vi "OAT Get Even Angle Reference (N Channels).vi"(0 "scaled signals [EU]":waveform(dbl)[](array[waveform]), 1 "reference output mode":T2(ring), 2 "reset? (F)":bool, 5 "speed profile":T1 {"speed [RPM]" format="%.2f"; "time [s]" format="%.2f"}, 7 "pulse/revolution (1)":i32=1, 9 "# of revs in reference":i32=1, 11 "error in (no error)":errorcluster, 12 "max order (auto)":dbl, 13 "remove DC? (F)":bool) -> (4 "even-angle references":cluster{"r0":dbl, "dr":dbl, "Y":dbl[]}[](array[cluster]) {"r0" format="%.2p"; "dr" format="%.2p"; "Y" format="%.2f"}, 14 "actual max order":dbl, 15 "error out":errorcluster)   [LabVIEW 2017, in "SoundVib_RefDataProcess.lvlib"]
doc: "Computes the even-angle reference of the <B>scaled signal [EU]</B>. The output reference is the even-angle spaced signal with a constant number of samples per revolution. Wire data to the <B>scaled signal [EU]</B> input to determine the polymorphic instance to use or manually select the instance."
uses:
  <vilib>/addons/Sound and Vibration/Order Analysis/Referece Data Processing/SoundVib_RefDataProcess.lvlib
  <vilib>/addons/Sound and Vibration/Order Analysis/Tach Process/SubVIs/speed profile.ctl
  <vilib>/addons/_NISVFA/_Shared subVIs/Common/svc_Check for Waveform Parameter Continuity (no state).vi
  <vilib>/addons/_NISVFA/_Shared subVIs/Common/svc_Get SV Channel Info.vi
  <vilib>/addons/Sound and Vibration/Order Analysis/Utility/OAT AC DC Separation (N Channels).vi
  <vilib>/addons/Sound and Vibration/Order Analysis/Resample Order Tracking/OAT Convert to Even Angle Signal (N Channels).vi
  <vilib>/addons/_NISVFA/_Shared subVIs/Common/svc_Engineering Units to Unit Label.vi
  <vilib>/addons/_NISVFA/_Shared subVIs/Common/svc_Unit Label to Engineering Units.vi
  <vilib>/addons/Sound and Vibration/Order Analysis/Resample Order Tracking/SoundVib_Resampling.lvlib
  <vilib>/addons/Sound and Vibration/Order Analysis/Resample Order Tracking/SoundVib_OrderTracking.lvlib
  <vilib>/addons/Sound and Vibration/Order Analysis/Utility/SoundVib_OAUtility.lvlib
  <vilib>/addons/Sound and Vibration/Order Analysis/Tach Process/SoundVib_TachProcess.lvlib
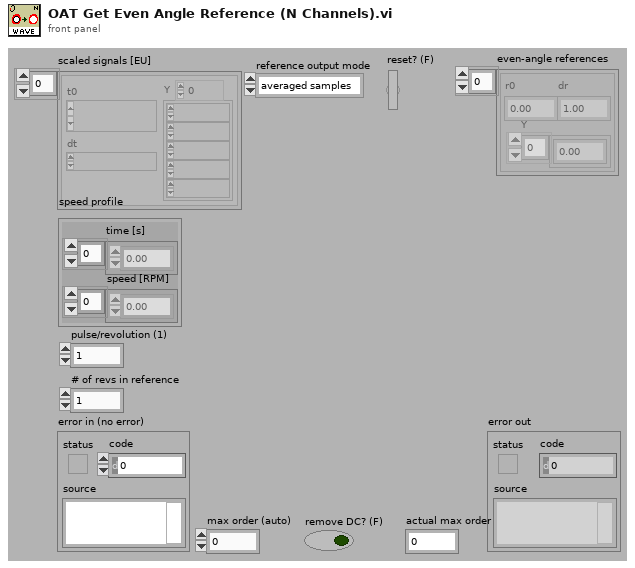
[diagram p1: front panel]
types:
  T1 = typedef "SoundVib_TachProcess.lvlib/speed profile.ctl" = cluster{"time [s]":dbl[], "speed [RPM]":dbl[]}
  T2 = enum16{"averaged samples", "initial samples", "final samples"}
  T3 = cluster{"dt equal":bool, "array length equal":bool, "number channels change":bool}
  T4 = cluster{"dt":bool, "t0 continuity":bool, "array length":bool, "channel info":bool, "name":bool}
  T5 = cluster{"r0":dbl, "dr":dbl, "reference data":dbl[]}[]
  T6 = typedef "svc_Resampled Channel Info.ctl" = cluster{"channel name":string, "description":string, " channel info":T7}
  T7 = typedef "svc_Channel Info.ctl" = cluster{"sensor sensitivity":dbl, "engineering units":T8, "dB reference":dbl, "custom label":string, "weighting filter":T9, "pregain":dbl}
  T8 = typedef "svc_Engineering Units Text Ring.ctl" = u16
  T9 = typedef "svc_Weighting Filter Text Ring.ctl" = u16
  T10 = typedef "OAT Position Info.ctl" = cluster{"positions [s]":dbl[], "samples/rev":dbl}
  T11 = cluster{"r0":dbl, "dr":dbl, "reference data":dbl[]}
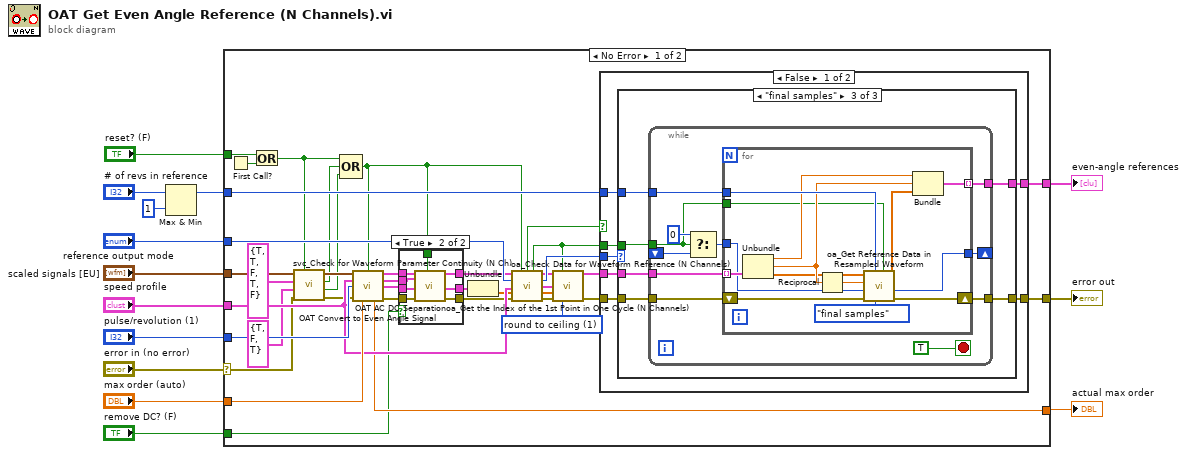
[diagram p0: block diagram]
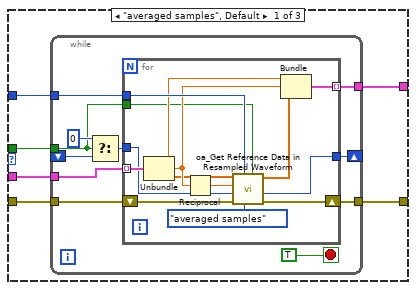
[diagram p3: hidden frame]
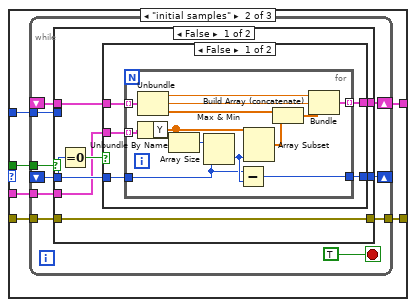
[diagram p4: hidden frame]
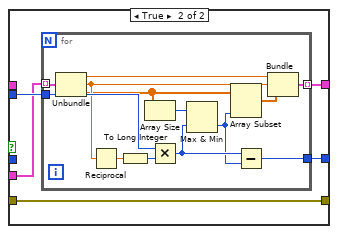
[diagram p6: hidden frame]
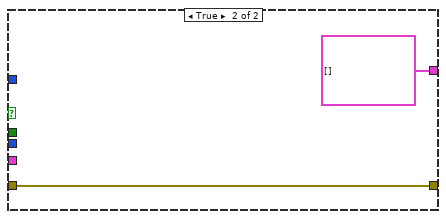
[diagram p7: hidden frame]
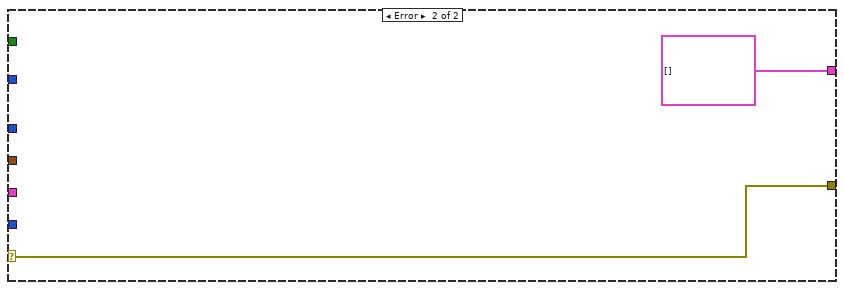
[diagram p8: hidden frame]
diagram:
  n1 = Max & Min(x="# of revs in reference", y=1) -> (max(x,y)=w9:i32)  [unwired: 1 out]
  n2 = case shown="No Error" "error in (no error)" {
    selector: "error in (no error)" -> [w22 w198]
    tunnel: "reference output mode" -> [w53 _]
    tunnel: [w52 T5 []] -> w12
    tunnel: [w51 w198] -> w11
    tunnel: w9 -> [w47 _]
    tunnel: "scaled signals [EU]" -> [w24 _]
    tunnel: "pulse/revolution (1)" -> [w44 _]
    tunnel: "max order (auto)" -> [w43 _]
    tunnel: "speed profile" -> [w42 _]
    tunnel: [w37 _] -> w3
    tunnel: "reset? (F)" -> [w36 _]
    tunnel: "remove DC? (F)" -> [w28 _]
    frame No Error {
      w33 = u16 1 items=["round to nearest", "round to ceiling"] ("index mode")
      n3 = First Call?() -> (First Call?: T/F=w38:bool)
      n4 = Or(x=w36, y=w38) -> (x .or. y?=w20:bool)
      n5 = call <vilib>:"svc_Check for Waveform Parameter Continuity (N Ch).vi"("restart averaging (F)"=w20, "error in (no error)"=w22, "checks for multichannel parameters"=T3 {"dt equal"=TRUE, "array length equal"=FALSE, "number channels change"=TRUE}, "checks for channel parameter change"=T4 {"dt"=TRUE, "t0 continuity"=TRUE, "array length"=FALSE, "channel info"=TRUE, "name"=FALSE}, "scaled signal(s)"=w24) -> ("error out"=w21:errorcluster, "multichannel parameter changed"=w17:bool, "waveform parameter changed"=w18:bool, "dup scaled signal(s)"=w23:waveform(dbl)[])  [unwired: 3 out]
      n6 = Compound Arithmetic op=OR(w20, w18, w17) -> (w19:bool)
      n7 = call-poly <vilib>:"OAT Convert to Even Angle Signal.vi"("scaled signals [EU]"=w23, "reset? (F)"=w19, "speed profile"=w42, "pulse/revolution (1)"=w44, "error in (no error)"=w21, "max order (auto)"=w43) -> ("even-angle signals"=w32:cluster{"r0":dbl, "dr":dbl, "Y":dbl[]}[], "even-angle channel info"=w29:T6[], "even-angle position info"=w26:T10, "actual max order"=w37:dbl, "error out"=w25:errorcluster)  [unwired: 5 in]
      n8 = case shown="True" w28 {
        tunnel: w32 -> [w56 w64]
        tunnel: [w56 w59] -> w31
        tunnel: w25 -> [w55 w63]
        tunnel: [w55 w62] -> w30
        tunnel: w19 -> [_ w61]
        tunnel: w29 -> [_ w60]
        tunnel: w26 -> [w54 w58]
        tunnel: [w54 w57] -> w27
        frame False {
        }
        frame True {
          n9 = call-poly <vilib>:"OAT AC DC Separation.vi"("even-angle signals"=w64, "even-angle channel info"=w60, "position info"=w58, "error in (no error)"=w63, "reset? (F)"=w61) -> ("even-angle AC signals"=w59:cluster{"r0":dbl, "dr":dbl, "Y":dbl[]}[], "position info out"=w57:T10, "error out"=w62:errorcluster)  [unwired: 9 in, 3 out]
        }
      }
      n10 = Unbundle(w27) -> ("positions [s]"=w39:dbl[])  [unwired: 1 out]
      n11 = call <vilib>:"oa_Check Data for Waveform Reference (N Channels).vi"("resampled signal"=w31, "reset? (True)"=w19, "select reference data"=w53, "speed profile"=w42, "interpolated pulse positions"=w39, "error in (no error)"=w30) -> ("empty signal?"=w35:bool, "reset"=w34:bool, "resampled data out"=w46:cluster{"r0":dbl, "dr":dbl, "Y":dbl[]}[], "select reference dataout"=w50:T2, "speed profile out"=w49:T1, "interpolated pulse positions out"=w48:dbl[], "error out"=w45:errorcluster)  [unwired: 2 in, 1 out]
      n12 = call <vilib>:"oa_Get the Index of the 1st Point in One Cycle (N Channels).vi"("resampled signal"=w46, "reset? (True)"=w34, "speed profile"=w49, "interpolated pulse positions"=w48, "error in (no error)"=w45, "index mode"=w33) -> ("resampled signal out"=w40:cluster{"r0":dbl, "dr":dbl, "Y":dbl[]}[], "error out"=w41:errorcluster)  [unwired: 7 in, 1 out]
      n13 = case shown="False" w35 {
        tunnel: [w71 T5 []] -> w52
        tunnel: [w70 w196] -> w51
        tunnel: w34 -> [w69 _]
        tunnel: w50 -> [w68 _]
        tunnel: w47 -> [w67 _]
        tunnel: w41 -> [w66 w196]
        tunnel: w40 -> [w65 _]
        frame False {
          n14 = case shown="\"final samples\"" w68 {
            tunnel: w69 -> [w77 w108 w169]
            tunnel: w67 -> [w76 w107 w168]
            tunnel: [w75 w105 w166] -> w71
            tunnel: [w74 w106 w167] -> w70
            tunnel: w66 -> [w72 w104 w165]
            tunnel: w65 -> [w73 w103 w164]
            frame "averaged samples", Default {
              n15 = while {
                tunnel: w77 -> [w79]
                tunnel: w76 -> [w87]
                tunnel: [w86] -> w75
                shift-right: [w85] -> _
                shift-left: _ -> [w83]
                tunnel: [w84] -> w74
                tunnel: w73 -> [w80]
                tunnel: w72 -> [w78]
                stop <- TRUE stop-if-true
                n16 = Select(t=0, s=w79, f=w83) -> (s? t:f=w81:i32)
                n17 = for {
                  tunnel: w80 -> [w92] mode=indexing
                  tunnel: w87 -> [w102]
                  tunnel: [w98] -> w86 mode=indexing
                  tunnel: [w97] -> w85
                  shift-right: [w96] -> w84
                  shift-left: w78 -> [w101]
                  tunnel: w81 -> [w90]
                  tunnel: w79 -> [w89]
                  n18 = Unbundle(w92) -> ("r0"=w94:dbl, "dr"=w93:dbl, "Y"=w91:dbl[])
                  n19 = Reciprocal(x=w93) -> (1/x=w99:dbl)
                  n20 = call <vilib>:"oa_Get Reference Data in Resampled Waveform.vi"("reset? (True)"=w89, "select reference data"=T2."averaged samples", "# of revs in reference data"=w102, "error in (no error)"=w101, "last index"=w90, "pulse per rev"=w99, "Y"=w91) -> ("error out"=w96:errorcluster, "last index out"=w97:i32, "reference data"=w100:dbl[])  [unwired: 2 in]
                  n21 = Bundle("r0"=w94, "dr"=w93, "reference data"=w100) -> (w98:T11)  [unwired: 1 in]
                }
              }
            }
            frame "initial samples" {
              n22 = while {
                tunnel: w108 -> [w111]
                tunnel: w107 -> [w117]
                shift-right: [w116] -> w105
                shift-left: _ -> [w114]
                shift-right: [w115] -> _
                shift-left: _ -> [w113]
                tunnel: [w112] -> w106
                tunnel: w104 -> [w110]
                tunnel: w103 -> [w109]
                stop <- TRUE stop-if-true
                n23 = case shown="False" w111 {
                  tunnel: w110 -> [w120 w146]
                  tunnel: w117 -> [_ w150]
                  tunnel: [w121 w149] -> w116
                  tunnel: [w125 w148] -> w115
                  tunnel: w114 -> [w124 _]
                  tunnel: w113 -> [w123 _]
                  tunnel: [w120 w146] -> w112
                  tunnel: w109 -> [w119 w147]
                  frame False {
                    n24 = Equal To 0?(x=w123) -> (x = 0?=w122:bool)
                    n25 = case shown="False" w122 {
                      tunnel: [w130 w144] -> w125
                      tunnel: w124 -> [w129 w145]
                      tunnel: w123 -> [w128 w144]
                      tunnel: [w127 w145] -> w121
                      tunnel: w119 -> [w126 _]
                      frame False {
                        n26 = for {
                          tunnel: [w142] -> w130
                          tunnel: w129 -> [w140] mode=indexing
                          tunnel: w128 -> [w139]
                          tunnel: [w134] -> w127 mode=indexing
                          tunnel: w126 -> [w133] mode=indexing
                          n27 = Unbundle(w140) -> ("r0"=w135:dbl, "dr"=w136:dbl, w132:dbl[])
                          n28 = Unbundle By Name(w133) -> ("Y"=w131:dbl[])
                          n29 = Array Size(array=w131) -> (size(s)=w143:i32)
                          n30 = Max & Min(x=w143, y=w139) -> (min(x,y)=w141:i32)  [unwired: 1 out]
                          n31 = Subtract(x=w139, y=w141) -> (x-y=w142:i32)
                          n32 = Array Subset(array=w131, length=w141) -> (w138:dbl[])  [unwired: 1 in]
                          n33 = Build Array (concatenate)(w132, w138) -> (w137:dbl[])
                          n34 = Bundle("r0"=w135, "dr"=w136, w137) -> (w134:cluster{"r0":dbl, "dr":dbl, dbl[]})  [unwired: 1 in]
                        }
                      }
                      frame True {
                      }
                    }
                  }
                  frame True {
                    n35 = for {
                      tunnel: w150 -> [w163]
                      tunnel: [w156] -> w149 mode=indexing
                      tunnel: [w155] -> w148
                      tunnel: w147 -> [w154] mode=indexing
                      n36 = Unbundle(w154) -> ("r0"=w153:dbl, "dr"=w152:dbl, "Y"=w151:dbl[])
                      n37 = Reciprocal(x=w152) -> (1/x=w162:dbl)
                      n38 = To Long Integer(number=w162) -> (32bit integer=w161:i32)
                      n39 = Array Size(array=w151) -> (size(s)=w160:i32)
                      n40 = Multiply(x=w163, y=w161) -> (x*y=w159:i32)
                      n41 = Max & Min(x=w160, y=w159) -> (min(x,y)=w158:i32)  [unwired: 1 out]
                      n42 = Array Subset(array=w151, length=w158) -> (w157:dbl[])  [unwired: 1 in]
                      n43 = Subtract(x=w159, y=w158) -> (x-y=w155:i32)
                      n44 = Bundle("r0"=w153, "dr"=w152, w157) -> (w156:cluster{"r0":dbl, "dr":dbl, dbl[]})  [unwired: 1 in]
                    }
                  }
                }
              }
            }
            frame "final samples" {
              n45 = while {
                tunnel: w169 -> [w170]
                tunnel: w168 -> [w179]
                tunnel: [w178] -> w166
                shift-right: [w177] -> _
                shift-left: _ -> [w175]
                tunnel: [w176] -> w167
                tunnel: w165 -> [w172]
                tunnel: w164 -> [w171]
                stop <- TRUE stop-if-true
                n46 = Select(t=0, s=w170, f=w175) -> (s? t:f=w173:i32)
                n47 = for {
                  tunnel: w179 -> [w194]
                  tunnel: [w190] -> w178 mode=indexing
                  tunnel: [w189] -> w177
                  tunnel: w171 -> [w186] mode=indexing
                  shift-right: [w188] -> w176
                  shift-left: w172 -> [w193]
                  tunnel: w173 -> [w182]
                  tunnel: w170 -> [w181]
                  n48 = Unbundle(w186) -> ("r0"=w185:dbl, "dr"=w184:dbl, "Y"=w183:dbl[])
                  n49 = Reciprocal(x=w184) -> (1/x=w191:dbl)
                  n50 = call <vilib>:"oa_Get Reference Data in Resampled Waveform.vi"("reset? (True)"=w181, "select reference data"=T2."final samples", "# of revs in reference data"=w194, "error in (no error)"=w193, "last index"=w182, "pulse per rev"=w191, "Y"=w183) -> ("error out"=w188:errorcluster, "last index out"=w189:i32, "reference data"=w192:dbl[])  [unwired: 2 in]
                  n51 = Bundle("r0"=w185, "dr"=w184, "reference data"=w192) -> (w190:T11)  [unwired: 1 in]
                }
              }
            }
          }
        }
        frame True {
        }
      }
    }
    frame Error {
    }
  }
  "error out" <- w11
  "even-angle references" <- w12
  "actual max order" <- w3
